vi "read gain full vi.vi"() -> ()   [LabVIEW 2009]
panel:
  out "result string":string
  out "VISA resource name out":refnum<visa-resource-name>
  in  "VISA resource name":refnum<visa-resource-name>="GPIB0::12::INSTR"
  in  "error in (no error)":errorcluster
  out "read buffer":string
  in  "read? (f)":bool=TRUE
  in  "bytes to read (1000)":u32=1000
  out "bytes read":u32
  out "error out":errorcluster
  in  "write buffer":string="RDA"
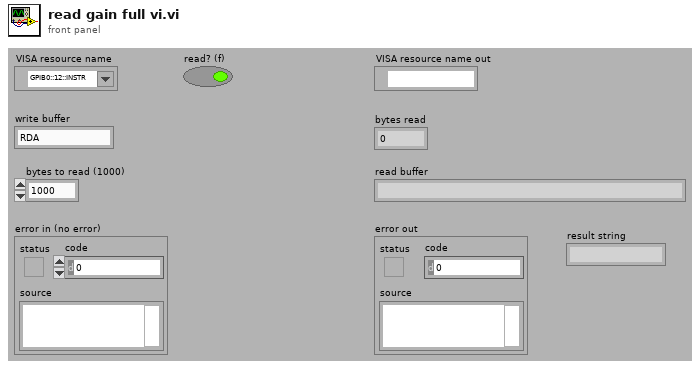
[diagram p1: front panel]
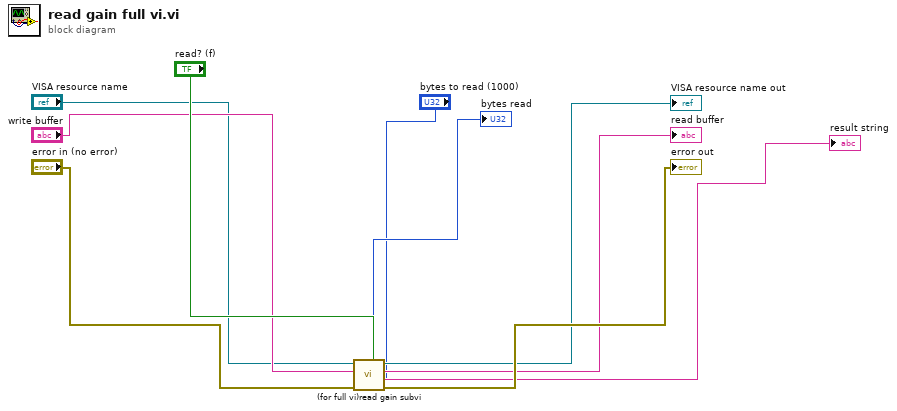
[diagram p0: block diagram]
diagram:
  n1 = call "(for full vi)read gain subvi.vi"("VISA resource name"="VISA resource name", "write buffer"="write buffer", "bytes to read (1000)"="bytes to read (1000)", "error in (no error)"="error in (no error)", "read? (f)"="read? (f)") -> ("bytes read"=→"bytes read":u32, "VISA resource name out"=→"VISA resource name out":refnum<visa-resource-name>, "read buffer"=→"read buffer":string, "result string"=→"result string":string, "error out"=→"error out":errorcluster)
